vi "get XY center and angle.vi"(9 "output P1 XY":bool, 11 "controller in":T1) -> (0 "XY theta out":dbl, 1 "XY center out":dbl[](array[numeric]), 3 "controller out":T1, 4 "offset P1-P2":dbl[](array[numeric]))   [LabVIEW 2016]
uses:
  Classes/Controller/Motion/A3200 Folder/A3200.lvclass
  Classes/Controller/Dispenser/Ultimus V2 Folder/Ultimus V2.lvclass
  Classes/Controller/I-O/NI-DAQ Folder/NI-DAQ.lvclass
  Classes/Controller/Motion/Motion Folder/Motion.lvclass
  Classes/Controller/I-O/I-O Folder/I-O.lvclass
  Classes/Controller/Dispenser/Dispenser Folder/Dispenser.lvclass
panel:
  in  "get P2":bool
  in  "get P1":bool
  out "P2":dbl[](array[numeric])=[1219.30639899585, 722.8896830877354, 52.864847366341415, 0.003106741190800654] format="%#_8g"
  out "P1":dbl[](array[numeric])=[1219.30639899585, 722.8896830877354, 52.864847366341415, 0.003106741190800654] format="%#_8g"
  out "Sum":dbl[](array[numeric])=[1219.30639899585, 722.8896830877354, 52.864847366341415, 0.003106741190800654] format="%#_8g"
  out "angle":dbl
  in  "start":bool
  in  "stop":bool
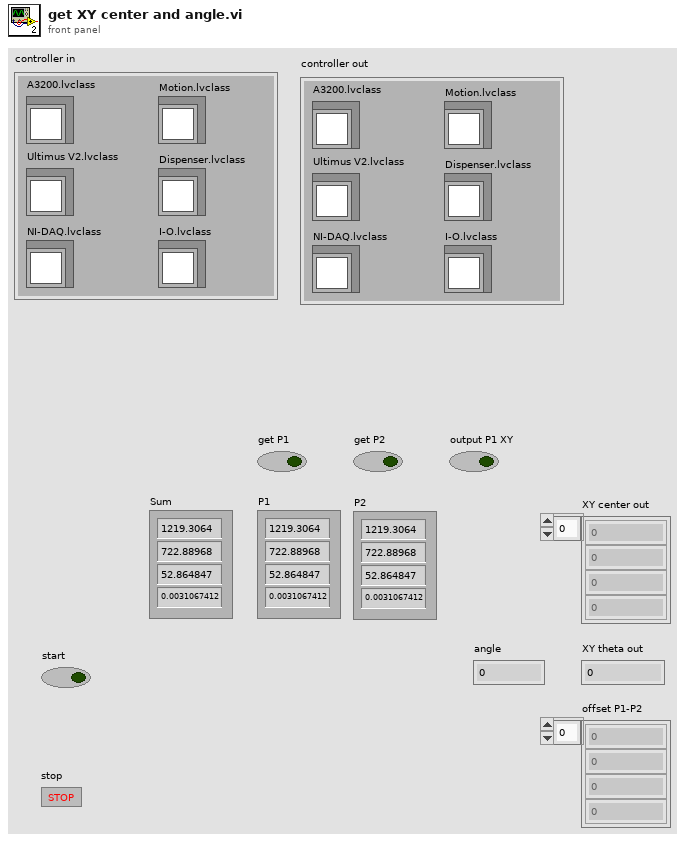
[diagram p1: front panel]
types:
  T1 = cluster{"A3200.lvclass":refnum<class "A3200.lvclass">, "Ultimus V2.lvclass":refnum<class "Ultimus V2.lvclass">, "NI-DAQ.lvclass":refnum<class "NI-DAQ.lvclass">, "Motion.lvclass":refnum<class "Motion.lvclass">, "I-O.lvclass":refnum<class "I-O.lvclass">, "Dispenser.lvclass":refnum<class "Dispenser.lvclass">}
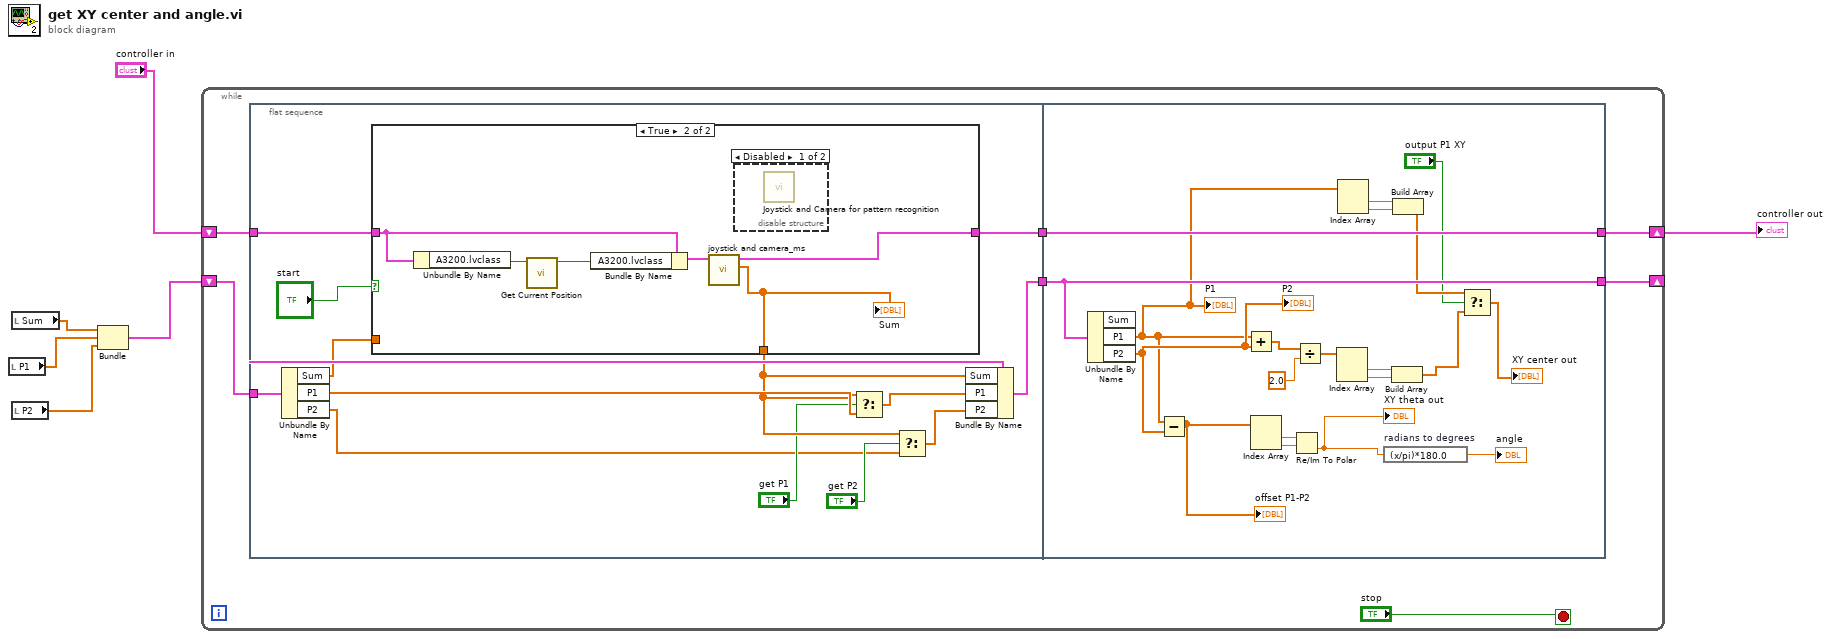
[diagram p0: block diagram]
diagram:
  n1 = local read "P1"() -> (w5:dbl[])
  n2 = local read "Sum"() -> (w6:dbl[])
  n3 = local read "P2"() -> (w4:dbl[])
  n4 = Bundle("Sum"=w6, "P1"=w5, "P2"=w4) -> (w3:cluster{"Sum":dbl[], "P1":dbl[], "P2":dbl[]})  [unwired: 1 in]
  n5 = while {
    shift-right: [w12] -> w2
    shift-left: "controller in" -> [w13]
    shift-right: [w7] -> _
    shift-left: w3 -> [w10]
    stop <- "stop" stop-if-true
    n6 = flat-sequence {
      tunnel: w13 -> [w26]
      tunnel: w10 -> [w24]
      tunnel: [w25] -> w9
      tunnel: [w14] -> w8
      tunnel: [w54] -> w12
      tunnel: w9 -> [w54]
      tunnel: w8 -> [w53]
      tunnel: [w53] -> w7
      frame #0 {
        n7 = Unbundle By Name(w24) -> ("Sum"=w22:dbl[], "P1"=w21:dbl[], "P2"=w15:dbl[])
        n8 = case shown="True" "start" {
          tunnel: w26 -> [w28 w33]
          tunnel: [w28 w29] -> w25
          tunnel: [w27 w31] -> w20
          tunnel: w22 -> [w27 _]
          frame False {
          }
          frame True {
            n9 = Unbundle By Name(w33) -> ("A3200.lvclass"=w34:refnum<class "A3200.lvclass">)
            n10 = call-dynamic "Get Current Position.vi"("Gantry in"=w34) -> ("Gantry out"=w32:refnum<class "A3200.lvclass">)  [unwired: 8 in, 2 out]
            n11 = Bundle By Name(cluster=w33, "A3200.lvclass"=w32) -> (w30:T1)
            n12 = call "joystick and camera_ms.vi"("controller in"=w30) -> ("Gantry"=w31:dbl[], "controller out"=w29:T1)  [unwired: 9 in]
            "Sum" <- w31
            n13 = disable-structure shown="Disabled" {
              frame Disabled {
                n14 = call "Joystick and Camera for pattern recognition.vi"() -> ()  [unwired: 8 in, 4 out]
              }
              frame Enabled {
              }
            }
          }
        }
        n15 = Select(t=w20, s="get P1", f=w21) -> (s? t:f=w19:dbl[])
        n16 = Select(t=w20, s="get P2", f=w15) -> (s? t:f=w18:dbl[])
        n17 = Bundle By Name(cluster=w24, "Sum"=w20, "P1"=w19, "P2"=w18) -> (w14:cluster{"Sum":dbl[], "P1":dbl[], "P2":dbl[]})
      }
      frame #1 {
        n18 = Unbundle By Name(w53) -> ("P1"=w41:dbl[], "P2"=w44:dbl[])  [unwired: 1 out]
        "P1" <- w41
        "P2" <- w44
        n19 = Subtract(x=w41, y=w44) -> (x-y=w43:dbl[])
        "offset P1-P2" <- w43
        n20 = Add(x=w41, y=w44) -> (x+y=w51:dbl[])
        n21 = Index Array(array=w43) -> (element #1=w46:dbl, element #2=w45:dbl)  [unwired: 2 in]
        n22 = Re/Im To Polar(2:w45, 3:w46) -> (0:w35:dbl)  [unwired: 1 out]
        "XY theta out" <- w35
        n23 = Divide(x=w51, y=2.0) -> (x/y=w48:dbl[])
        n24 = Index Array(array=w48) -> (element #1=w49:dbl, element #2=w50:dbl)  [unwired: 2 in]
        n25 = Index Array(array=w41) -> (element #1=w42:dbl, element #2=w40:dbl)  [unwired: 2 in]
        n26 = expression code="(x/pi)*180.0" "radians to degrees"(w35) -> (→"angle":dbl)
        n27 = Build Array(w49, w50) -> (w39:dbl[])
        n28 = Build Array(w42, w40) -> (w37:dbl[])
        n29 = Select(t=w37, s="output P1 XY", f=w39) -> (s? t:f=→"XY center out":dbl[])
      }
    }
  }
  "controller out" <- w2
